vi "Event.vi"() -> ()   [LabVIEW 2018, in "ScratchpadLibrary.lvlib"]
uses:
  ScratchpadLibrary.lvlib
  <vilib>/event_ctls.llb/lveventtype.ctl
  <vilib>/event_ctls.llb/eventsource.ctl
panel:
  out "Interval":i64
  in  "Frequency":dbl(slide) scale=0.01..10.0
  out "Source":T1 items=["LabVIEW UI"=0, "ActiveX"=1, "User Event"=25]
  out "Type":T2=enum."Value Change"
  out "Timeout time":u32
  in  "Stop Button":bool
  out "Boolean 2":bool
  out "Boolean":bool
  out "Cycle":i32
  in  "Copy Button":bool
  in  "Add Button":bool
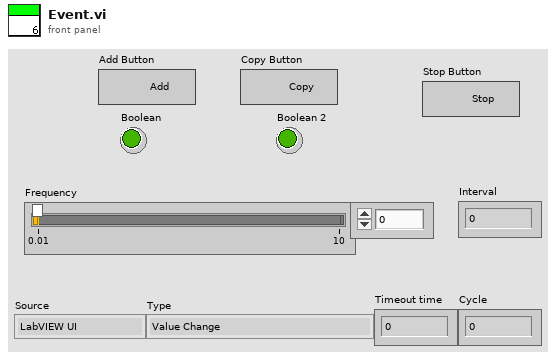
[diagram p1: front panel]
types:
  T1 = typedef "eventsource.ctl" = u32
  T2 = typedef "lveventtype.ctl" = enum32{"Null", "Timeout", "Annotation Menu Selection", "Annotation Menu Selection?", "App Instance Close", "App Instance Close?", "Autoscale Range Change", "Bookmark Info Change", "Cell Edit", "Cell Edit?", "Cursor Grab", "Cursor Grab?", "Cursor Menu Selection", "Cursor Menu Selection?", "Cursor Move", "Cursor Release", "Data Change", "Direction Change", "Display State Change", "Drag Ended", "Drag Enter", "Drag Leave", "Drag Over", "Drag Source Update", "Drag Starting", "Drag Starting?", "Drop", "Exec State Change", "Key Down", "Key Down?", "Key Repeat", "Key Repeat?", "Key Up", "Listbox Double Click", "Menu Activation?", "Menu Selection (App)", "Menu Selection? (App)", "Menu Selection (User)", "Mouse Down", "Mouse Down?", "Mouse Enter", "Mouse Leave", "Mouse Move", "Mouse Up", "Mouse Wheel", "NI Security User Change (App)", "Pane Size", "Panel Close", "Panel Close?", "Panel Resize", "Plot Attribute Change", "Scale Range Change", "Shortcut Menu Activation?", "Shortcut Menu Selection (App)", "Shortcut Menu Selection? (App)", "Shortcut Menu Selection (User)", "Tree Double Click", "Tree Drag", "Tree Drag?", "Tree Drop", "Tree Drop?", "Tree Item Close", "Tree Item Close?", "Tree Item Open", "Tree Item Open?", "User Event", "Value Change"}
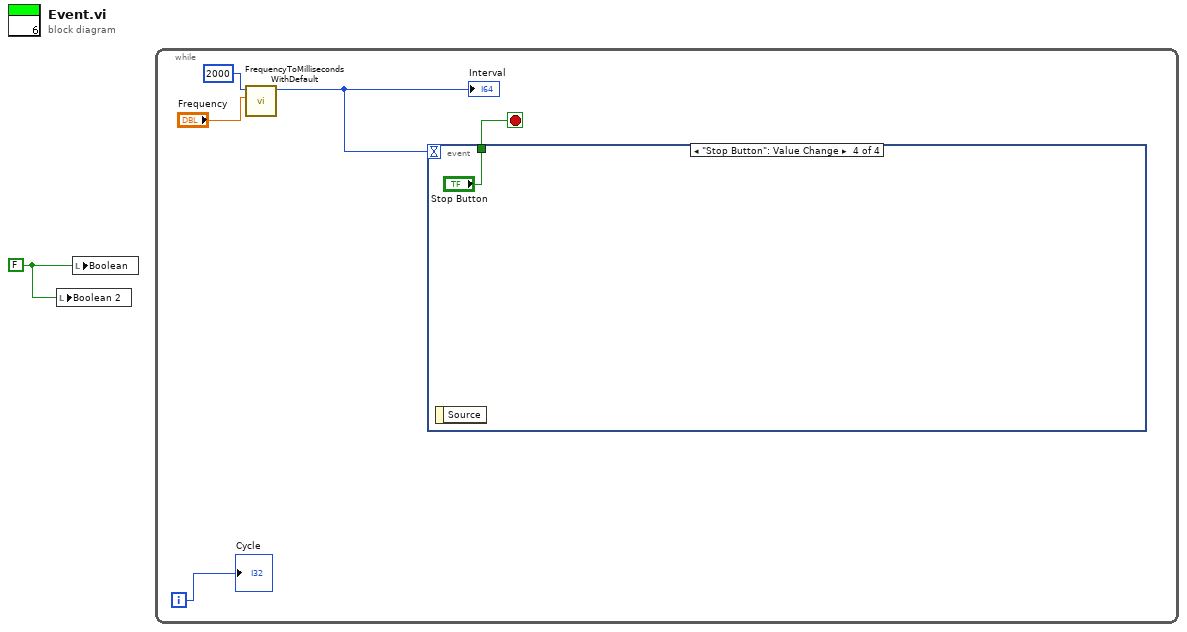
[diagram p0: block diagram]
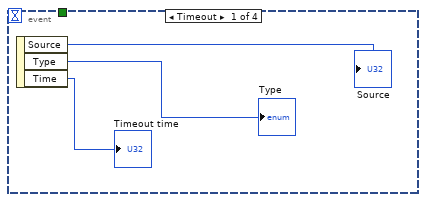
[diagram p2: hidden frame]
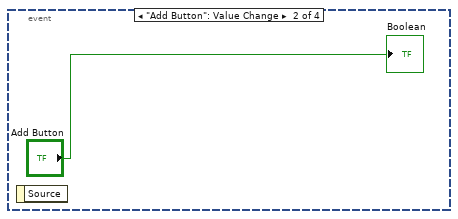
[diagram p3: hidden frame]
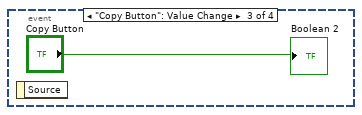
[diagram p4: hidden frame]
diagram:
  w1 = FALSE ("Boolean")
  n1 = local write "Boolean 2"(w1) -> ()
  n2 = local write "Boolean"(w1) -> ()
  n3 = while {
    i -> [w6]
    stop <- w3 stop-if-true
    n4 = call "FrequencyToMillisecondsWithDefault.vi"("Frequency"="Frequency", "Default in"=i64 2000) -> ("Default out"=w2:i64)  [unwired: 9 in]
    "Interval" <- w2
    n5 = event shown="[3] \"Stop Button\": Value Change" {
      selector: _ -> [_ _ _ _]
      dyn-events: _ -> [_ _ _ _]
      timeout: w2 -> [_ _ _ _]
      tunnel: [_ _ _ "Stop Button"] -> w3
      event Timeout {
        n6 = event-data() -> ("Source"=→"Source":T1, "Type"=→"Type":T2, "Time"=→"Timeout time":u32)  [unwired: 1 in]
      }
      event "Add Button": Value Change {
        n7 = event-data() -> ()  [unwired: 1 in, 1 out]
        "Boolean" <- "Add Button"
      }
      event "Copy Button": Value Change {
        n8 = event-data() -> ()  [unwired: 1 in, 1 out]
        "Boolean 2" <- "Copy Button"
      }
      event "Stop Button": Value Change {
        n9 = event-data() -> ()  [unwired: 1 in, 1 out]
      }
    }
    "Cycle" <- w6
  }
